vi "Receive.vi"(8 "error in (no error)":errorcluster caption="错误输入（无错误）", 10 "Receive":string, 11 "Custor 输入":refnum<class "Custor.lvclass">) -> (0 "error out":errorcluster caption="错误输出", 3 "Custor 输出":refnum<class "Custor.lvclass">)   [LabVIEW 2024, in "Custor.lvlib" / "Custor.lvclass"]
uses:
  Custor.lvclass
  <vilib>/ActorFramework/Actor/Actor.lvclass/Actor.ctl
  <vilib>/ActorFramework/Message Enqueuer/Message Enqueuer.lvclass/Message Enqueuer.ctl
  <vilib>/ActorFramework/Message Enqueuer/Enqueue.vi
  <vilib>/ActorFramework/Message Priority Queue/Priority Enqueue.vi
  Custor.lvclass/Custor.ctl
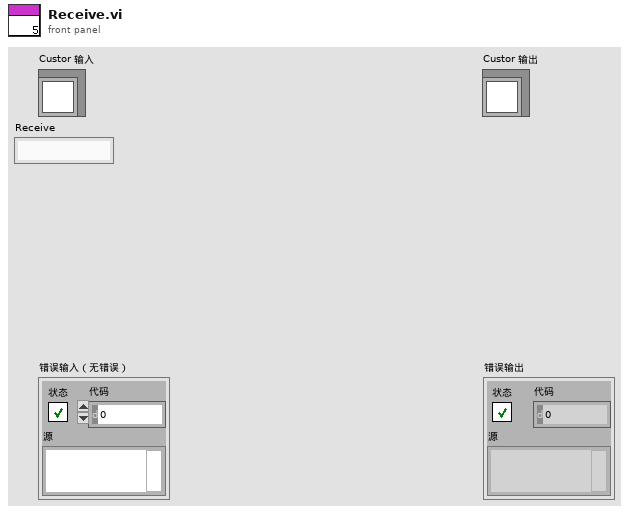
[diagram p1: front panel]
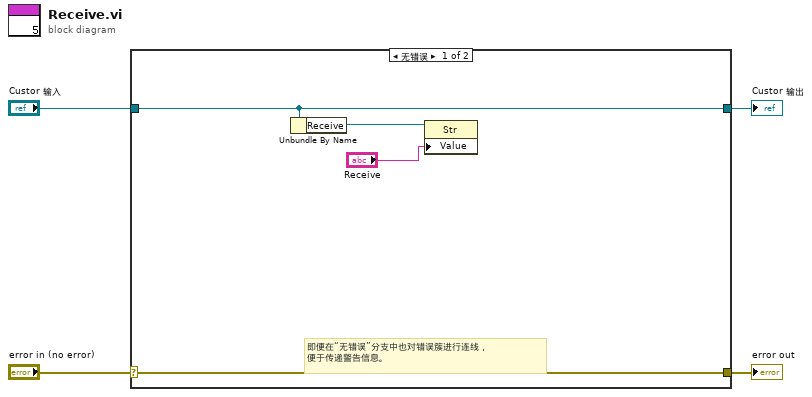
[diagram p0: block diagram]
diagram:
  n1 = case shown="无错误" "error in (no error)" {
    selector: "error in (no error)" -> [w8 w10]
    tunnel: [w8 w10] -> w3
    tunnel: [w7 w9] -> w1
    tunnel: "Custor 输入" -> [w7 w9]
    frame No Error {
      # "即便在“无错误”分支中也对错误簇进行连线，\n便于传递警告信息。"
      n2 = Unbundle By Name(w7) -> ("Receive"=w6:refnum<vi>)
      n3 = property class="Str"(reference=w6, "Value"="Receive") -> ()  [unwired: 1 in, 2 out]
    }
    frame Error {
    }
  }
  "error out" <- w3
  "Custor 输出" <- w1
